vi "Create Generic - 3 Queues.vi"(8 "error in (no error)":errorcluster, 11 "name":string="selectspectrum") -> (0 "error out":errorcluster, 3 "Message Queues":T1)   [LabVIEW 2023, in "Front Panel Message Queue.lvlib"]
doc: "This VI creates and initializes all the message queues for your application. If your application requires more than one message queue, right-click the \"Message Queues\" constant above and select Open Type Def. Add the new Message Queue(s) to the type definition, then initialize them in this VI."
uses:
  Front Panel Message Queue.lvlib
  load 3 Messages Queues.ctl
  Message Cluster.ctl
  Enqueue Message (Single).vi
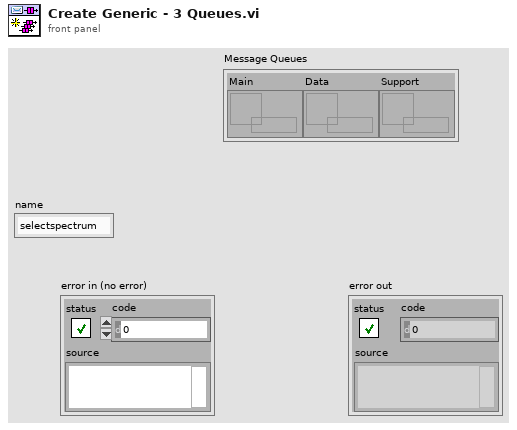
[diagram p1: front panel]
types:
  T1 = typedef "Front Panel Message Queue.lvlib/load 3 Messages Queues.ctl" = cluster{"Main":refnum<queue>, "Data":refnum<queue>, "Support":refnum<queue>}
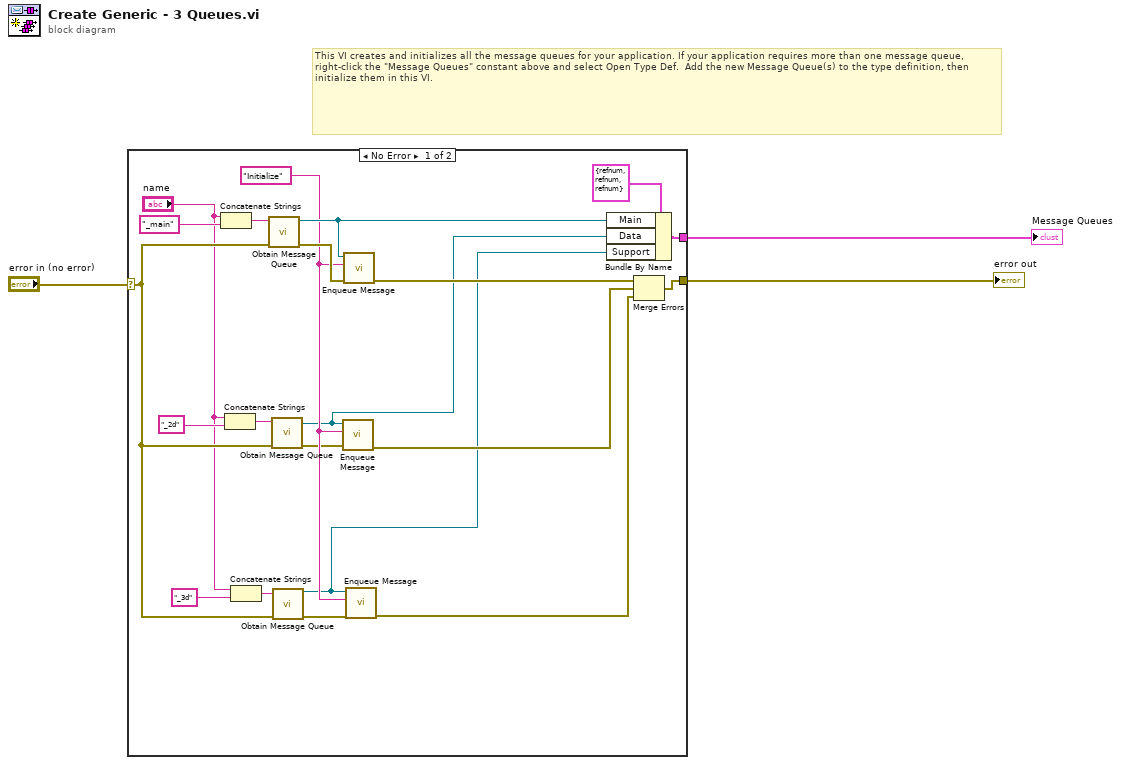
[diagram p0: block diagram]
diagram:
  # "This VI creates and initializes all the message queues for your application. If your application requires more than one message queue, right-click the \"Message Queues\" constant above and select Open Type Def.  Add the new Message Queue(s) to the type definition, then initialize them in this VI."
  n1 = case shown="No Error" "error in (no error)" {
    selector: "error in (no error)" -> [w17 w25]
    tunnel: [w20 w25] -> w3
    tunnel: [w24 _] -> w1
    frame No Error {
      w18 = "Initialize" ("Message")
      n2 = Concatenate Strings("name", "_main" ("Message")) -> (w10:string)
      n3 = Concatenate Strings("name", "_2d" ("Message")) -> (w8:string)
      n4 = Concatenate Strings("name", "_3d" ("Message")) -> (w7:string)
      n5 = call "Obtain Message Queue.vi"("error in (no error)"=w17, "name"=w10) -> ("error out"=w23:errorcluster, "Message Queue"=w22:refnum<queue>)  [unwired: 8 in]
      n6 = call "Obtain Message Queue.vi"("error in (no error)"=w17, "name"=w8) -> ("error out"=w15:errorcluster, "Message Queue"=w12:refnum<queue>)  [unwired: 8 in]
      n7 = call "Obtain Message Queue.vi"("error in (no error)"=w17, "name"=w7) -> ("error out"=w16:errorcluster, "Message Queue"=w11:refnum<queue>)  [unwired: 8 in]
      n8 = call-poly "Enqueue Message.vi"("error in (no error)"=w15, "Message"=w18, "Message Queue"=w12) -> ("error out"=w14:errorcluster)  [unwired: 7 in, 1 out]
      n9 = call-poly "Enqueue Message.vi"("error in (no error)"=w23, "Message"=w18, "Message Queue"=w22) -> ("error out"=w19:errorcluster)  [unwired: 7 in, 1 out]
      n10 = call-poly "Enqueue Message.vi"("error in (no error)"=w16, "Message"=w18, "Message Queue"=w11) -> ("error out"=w13:errorcluster)  [unwired: 7 in, 1 out]
      n11 = Bundle By Name(cluster=T1 {"Main"=refnum, "Data"=refnum, "Support"=refnum} ("Message Queues"), "Main"=w22, "Data"=w12, "Support"=w11) -> (w24:T1)
      n12 = Merge Errors(w19, w14, w13) -> (w20:errorcluster)
    }
    frame Error {
    }
  }
  "error out" <- w3
  "Message Queues" <- w1
